vi "Arduino-test-read.vi"() -> ()   [LabVIEW 2021]
uses:
  64700271-679b-4bb6-9256-cb1c1de197b1.vi
  9e36e6b7-9197-4346-99a9-fbc4c8936a64.vi
  c5256d6e-873c-4021-8c48-47191f8643cd.vi
  FW Arduino Control.lvclass
panel:
  in  "Command":string="Q0S"
  in  "baud rate (9600)":u32=115200
  in  "error in (no error)":errorcluster
  out "Array":u32[](array[numeric])
  out "reference out":refnum<visa-resource-name>
  out "error out":errorcluster
  in  "milliseconds to wait":u32=100
  out "response":string
  in  "Motor ID (0:n-1)":i32
  in  "VISA resource name":refnum<visa-resource-name>="COM9"
  # "Arduino standard baud rate: \n115200"
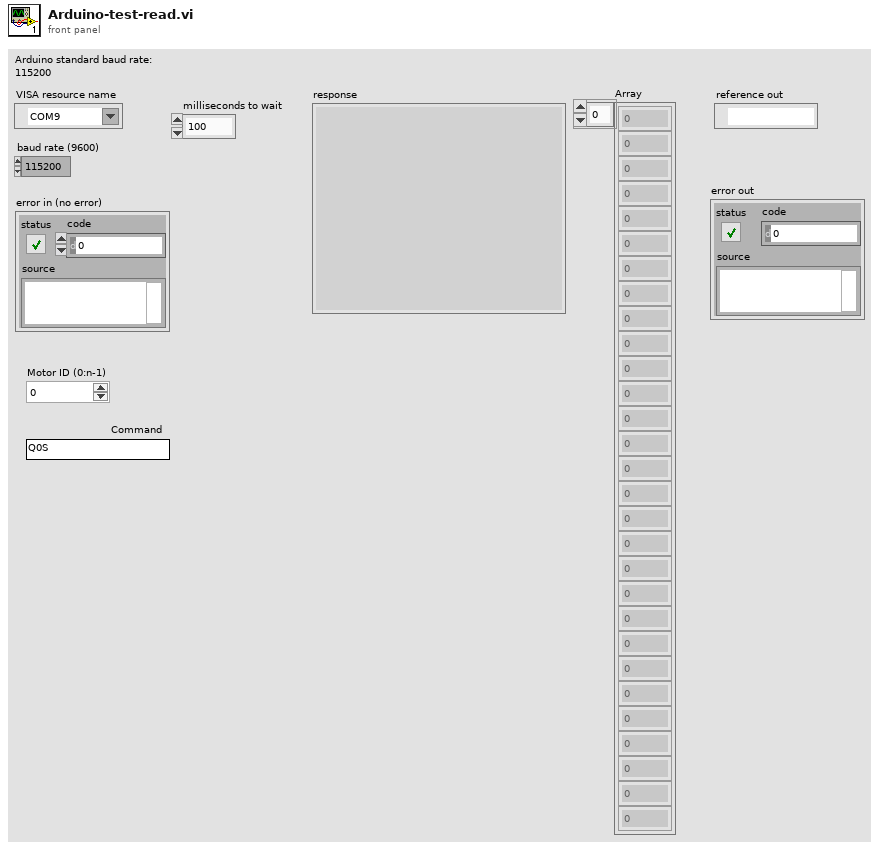
[diagram p1: front panel]
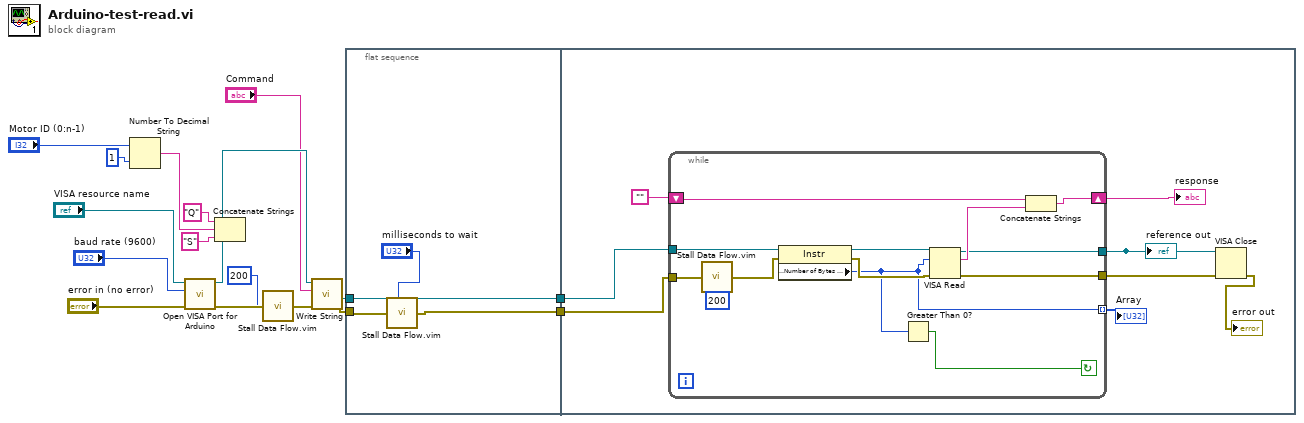
[diagram p0: block diagram]
diagram:
  n1 = Number To Decimal String(number="Motor ID (0:n-1)", width (-)=i16 1) -> (decimal integer string=w13:string)
  n2 = call "Open VISA Port for Arduino.vi"("error in (no error)"="error in (no error)", "baud rate (9600)"="baud rate (9600)", "VISA resource name"="VISA resource name") -> ("error out"=w4:errorcluster, "VISA resource name out"=w7:refnum<visa-resource-name>)  [unwired: 7 in]
  n3 = Concatenate Strings("Q", w13, "S") -> ()  [unwired: 1 out]
  n4 = call "Stall Data Flow.vim"("value in"=w4, "milliseconds to wait"=u32 200) -> ("value out"=w3:errorcluster)  [unwired: 1 out]
  n5 = call "Write String.vi"("error in (no error)"=w3, "String"="Command", "VISA resource name"=w7) -> ("error out"=w10:errorcluster, "VISA resource name out"=w14:refnum<visa-resource-name>)  [unwired: 7 in]
  n6 = flat-sequence {
    tunnel: w14 -> [w21]
    tunnel: [w21] -> w11
    tunnel: w10 -> [w20]
    tunnel: [w19] -> w9
    tunnel: w11 -> [w26]
    tunnel: w9 -> [w27]
    frame #0 {
      n7 = call "Stall Data Flow.vim"("value in"=w20, "milliseconds to wait"="milliseconds to wait") -> ("value out"=w19:errorcluster)  [unwired: 1 out]
    }
    frame #1 {
      n8 = while {
        tunnel: w26 -> [w42]
        tunnel: w27 -> [w40]
        shift-right: [w34] -> w28
        shift-left: "" -> [w35]
        tunnel: [w33] -> w24
        tunnel: [w32] -> w23
        tunnel: [w31] -> w25 mode=indexing
        stop <- w30 continue-if-true
        n9 = call "Stall Data Flow.vim"("value in"=w40, "milliseconds to wait"=u32 200) -> ("value out"=w39:errorcluster)  [unwired: 1 out]
        n10 = property class="Instr"(reference=w42, error in=w39) -> (reference out=w41:refnum<visa-resource-name>, error out=w37:errorcluster, "Serial Settings:Number of Bytes at Serial Port"=w31:u32)
        n11 = Greater Than 0?(x=w31) -> (x > 0?=w30:bool)
        n12 = VISA Read(VISA resource name=w41, byte count=w31, error in (no error)=w37) -> (VISA resource name out=w33:refnum<visa-resource-name>, read buffer=w36:string, error out=w32:errorcluster)  [unwired: 1 out]
        n13 = Concatenate Strings(w35, w36) -> (w34:string)
      }
      "response" <- w28
      "reference out" <- w24
      "Array" <- w25
      n14 = VISA Close(VISA resource name=w24, error in (no error)=w23) -> (error out=→"error out":errorcluster)
    }
  }
